vi "publish -- init -- 5.vi"(7 "publisher action":T1) -> (0 "request event":refnum<user-event>, 1 "response event":refnum<user-event>)   [LabVIEW 2018]
uses:
  publisher action.ctl
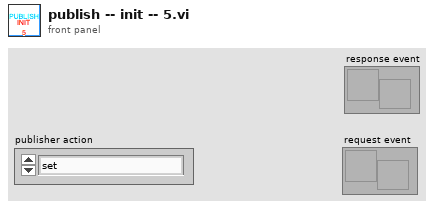
[diagram p1: front panel]
types:
  T1 = typedef "publisher action.ctl" = enum16{"set", "get", "init", "check"}
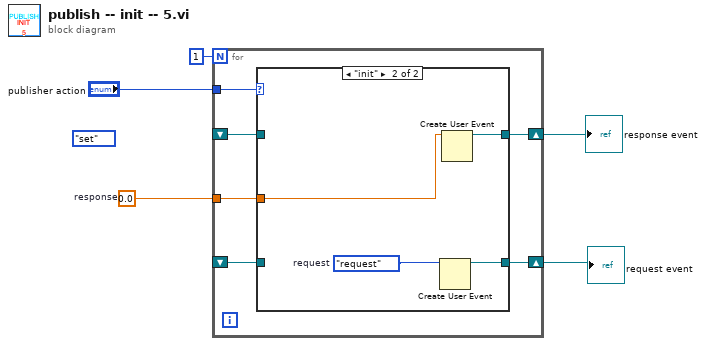
[diagram p0: block diagram]
diagram:
  w1 = 0.0  # response
  (unwired) publisher_action."set" ("publisher action")
  n1 = for {
    N: 1 -> [_]
    shift-right: [w11] -> w5
    shift-left: _ -> [w7]
    shift-right: [w10] -> w4
    shift-left: _ -> [w8]
    tunnel: "publisher action" -> [w9]
    tunnel: w1 -> [w6]
    n2 = case shown="\"init\"" w9 {
      tunnel: [w12 w16] -> w11
      tunnel: [w13 w15] -> w10
      tunnel: w8 -> [w13 _]
      tunnel: w7 -> [w12 _]
      tunnel: w6 -> [_ w14]
      frame "check", Default {
      }
      frame "init" {
        w17 = enum16{"request"}."request"  # request
        n3 = Create User Event(user event datatype=w17) -> (user event=w16:refnum<user-event>)  [unwired: 1 in, 1 out]
        n4 = Create User Event(user event datatype=w14) -> (user event=w15:refnum<user-event>)  [unwired: 1 in, 1 out]
      }
    }
  }
  "response event" <- w4
  "request event" <- w5
